vi "Movimiento nanometrico XYZ SIN CICLO.vi"(1 "Micras":bool, 2 "Stop Button":bool, 3 "Error In":errorcluster, 4 "Movimiento en Z":dbl min=0.0 max=100.0 format="%#_7g", 5 "Movimiento en Y":dbl min=0.0 max=100.0 format="%#_7g", 6 "Movimiento en X":dbl min=0.0 max=100.0 format="%#_7g") -> (0 "Error Out":errorcluster)   [LabVIEW 2018]
panel:
  # "El movimiento maximo del sistema son 100 Micrometros"
  # "Nanometros"
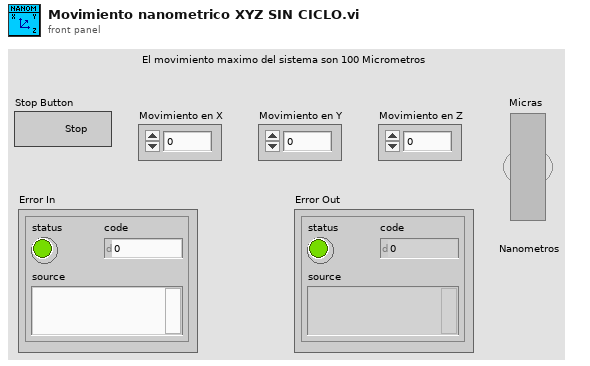
[diagram p1: front panel]
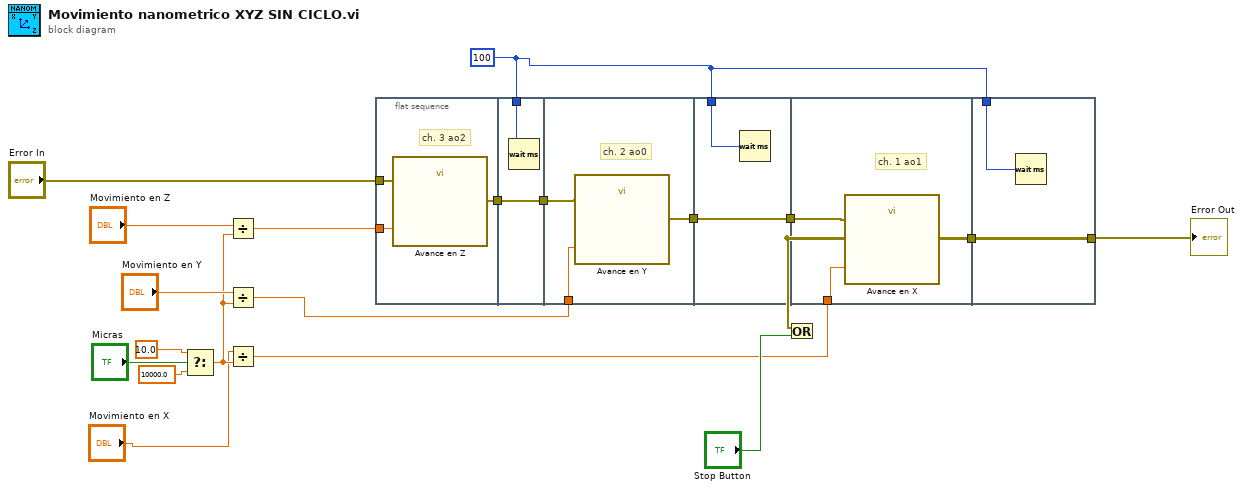
[diagram p0: block diagram]
diagram:
  w1 = 100
  n1 = Select(t=10.0 ("y"), s="Micras", f=10000.0 ("y")) -> (s? t:f=w14:dbl)
  n2 = Divide(x="Movimiento en Z", y=w14) -> (x/y=w9:dbl)
  n3 = Divide(x="Movimiento en Y", y=w14) -> (x/y=w7:dbl)
  n4 = Divide(x="Movimiento en X", y=w14) -> (x/y=w10:dbl)
  n5 = flat-sequence {
    tunnel: w9 -> [w22]
    tunnel: "Error In" -> [w21]
    tunnel: [w20] -> w6
    tunnel: w6 -> [w24]
    tunnel: [w24] -> w5
    tunnel: w1 -> [w23]
    tunnel: [w27] -> w4
    tunnel: w5 -> [w26]
    tunnel: w7 -> [w25]
    tunnel: w4 -> [w29]
    tunnel: [w29] -> w3
    tunnel: w1 -> [w28]
    tunnel: w10 -> [w30]
    tunnel: w3 -> [w31]
    tunnel: [w32] -> w2
    tunnel: [w34] -> w12
    tunnel: w2 -> [w34]
    tunnel: w1 -> [w33]
    frame #0 {
      # "ch. 3 ao2"
      n6 = call "Avance en Z"("data"=w22, "error in"=w21) -> ("error out"=w20:errorcluster)  [unwired: 16 in, 1 out]
    }
    frame #1 {
      n7 = Wait (ms)(milliseconds to wait=w23) -> ()  [unwired: 1 out]
    }
    frame #2 {
      # "ch. 2 ao0"
      n8 = call "Avance en Y"("data"=w25, "error in"=w26) -> ("error out"=w27:errorcluster)  [unwired: 16 in, 1 out]
    }
    frame #3 {
      n9 = Wait (ms)(milliseconds to wait=w28) -> ()  [unwired: 1 out]
    }
    frame #4 {
      # "ch. 1 ao1"
      n10 = call "Avance en X"("data"=w30, "error in"=w31) -> ("error out"=w32:errorcluster)  [unwired: 16 in, 1 out]
    }
    frame #5 {
      n11 = Wait (ms)(milliseconds to wait=w33) -> ()  [unwired: 1 out]
    }
  }
  n12 = Or(x=w12, y="Stop Button") -> ()  [unwired: 1 out]
  "Error Out" <- w12
